vi "All Values.vi"(8 "error in (no error)":errorcluster, 11 "Group in":refnum<class "Group.lvclass">) -> (0 "error out":errorcluster, 2 "Channel Value":T1[](array[typedef]) {"Timestamp" format="%<%H:%M:%S%3u>T"}, 3 "Group out":refnum<class "Group.lvclass">)   [LabVIEW 2020, in "Vecto.lvlib" / "Group.lvclass"]
uses:
  Group.lvclass
  Group.lvclass/Group.ctl
  Channel Value.ctl
  Vecto.lvlib
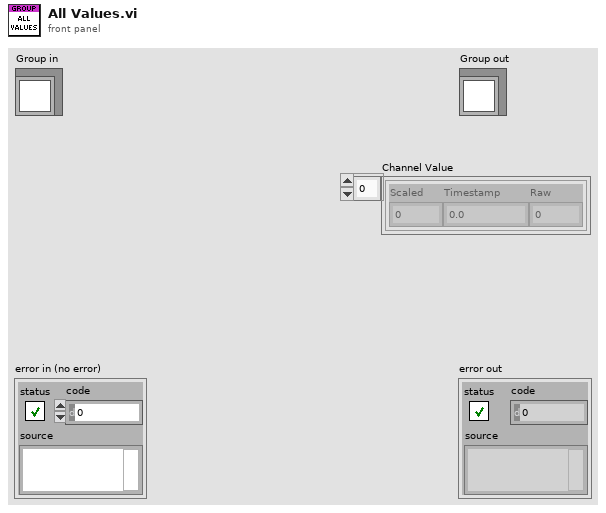
[diagram p1: front panel]
types:
  T1 = typedef "Vecto.lvlib/Channel Value.ctl" = cluster{"Scaled":dbl, "Timestamp":dbl, "Raw":dbl}
  T2 = typedef "Vecto.lvlib/Group.lvclass/Ref.ctl" = cluster{"Channel Index Map":map{string, i32}, "Channel Info":T3[], "Scaled":dbl[], "Timestamp":dbl[], "Raw":dbl[]}
  T3 = typedef "Vecto.lvlib/Channel Info.ctl" = cluster{"Name":string, "Group":string, "Owning Node":u32, "Owning Task":u32, "Resource":string}
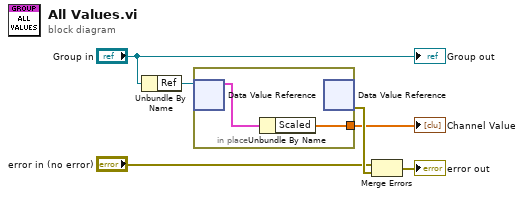
[diagram p0: block diagram]
diagram:
  n1 = Unbundle By Name("Group in") -> ("Ref"=w4:refnum<data-value>)
  n2 = in-place {
    in-place-border: [w7] -> w2
    n3 = in-place-dvr #1(w4) -> (w8:T2)  [unwired: 1 out]
    n4 = Unbundle By Name(w8) -> ("Scaled"=w7:dbl[])
    n5 = in-place-dvr #1() -> (w6:errorcluster)  [unwired: 1 in, 1 out]
  }
  "Channel Value" <- w2
  n6 = Merge Errors("error in (no error)", w6) -> (→"error out":errorcluster)
  "Group out" <- "Group in"
